vi "Subvi pixel clock.vi"(9 "Line clock":bool) -> (3 "Pixel clock/line clock change":cluster{"Pixel clock":bool, "Line clock":bool})   [LabVIEW 2017]
uses:
  GV N pixel clock per line.vi
  <vilib>/rvi/Memory/Memory_Emulation/nirvimemoryFastEmulation.vi
  <vilib>/rvi/Memory/Memory_Emulation/nirvimemoryEmulation.vi
  <vilib>/rvi/Emulation/niFpgaEmulationIsFPGAContextNoSignature.vi
  <vilib>/rvi/DataTransferAndStorage/Container/Common/niFpgaContainerGetUniqueNameForEmu.vi
  <vilib>/rvi/Emulation/niFpgaProcessEmulError.vi
  <vilib>/rvi/Emulation/niFpgaSctlEmulationGetInTimedLoop.vi
  <vilib>/rvi/errors/nirviReportUnexpectedCaseInternalError (U32).vi
  <vilib>/rvi/DataTransferAndStorage/Container/XNode/niFpgaContainer.xnode
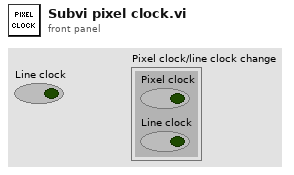
[diagram p1: front panel]
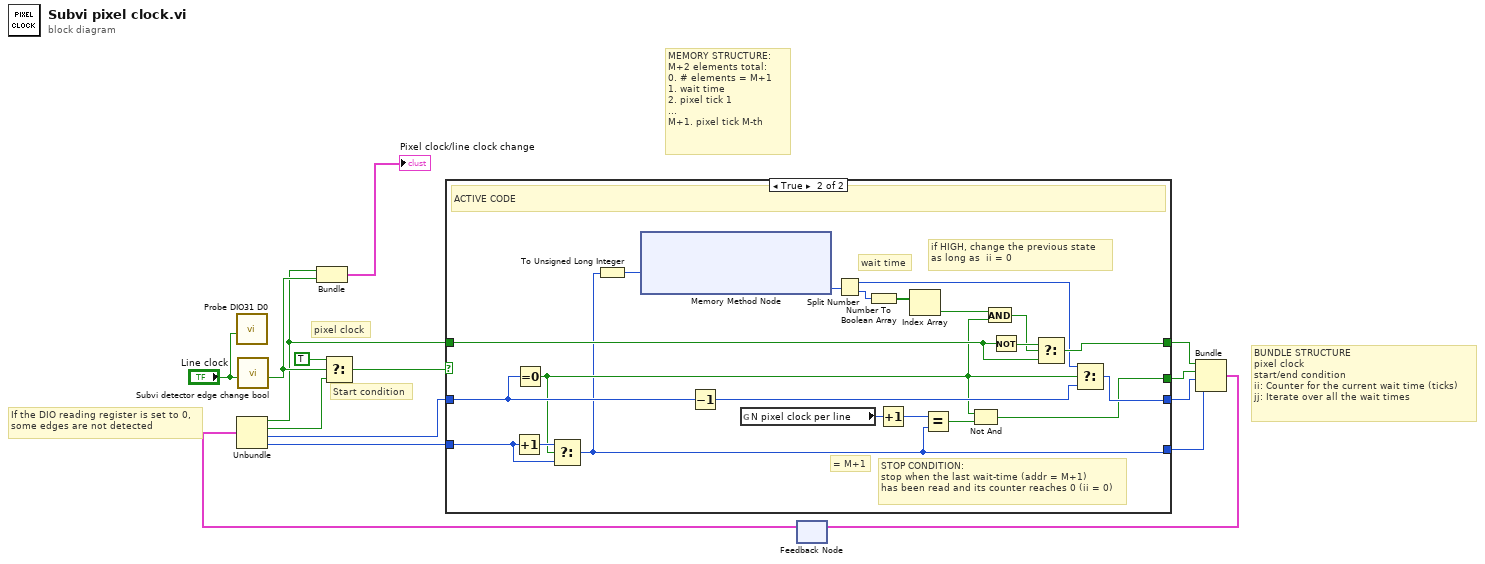
[diagram p0: block diagram]
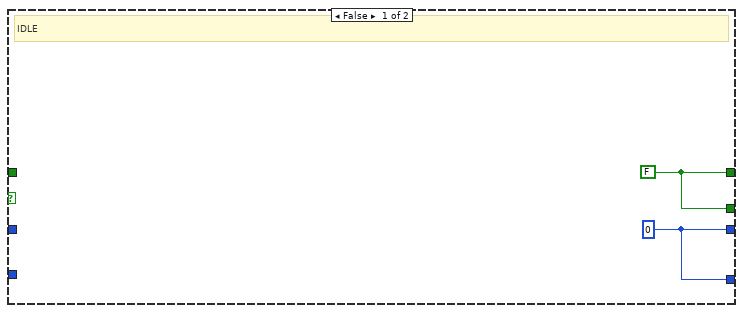
[diagram p2: hidden frame]
diagram:
  # "pixel clock"
  # "If the DIO reading register is set to 0,\nsome edges are not detected"
  # "BUNDLE STRUCTURE\npixel clock\nstart/end condition\nii: Counter for the current wait time (ticks)\njj: Iterate over all the wait times"
  # "MEMORY STRUCTURE:\nM+2 elements total:\n0. # elements = M+1\n1. wait time \n2. pixel tick 1\n...\nM+1. pixel tick M-th"
  # "Start condition"
  n1 = call "Probe DIO31 D0.vi"("D0"="Line clock") -> ()  [unwired: 11 in]
  n2 = call "Subvi detector edge change bool.vi"("Input"="Line clock") -> ("Output"=w3:bool)  [unwired: 8 in]
  n3 = feedback #1() -> (w8:cluster{bool, bool, u16, u16})  [unwired: 1 in]
  n4 = Unbundle(w8) -> (w1:bool, w6:bool, w5:u16, w4:u16)
  n5 = Bundle(w1, "Output"=w3) -> (→"Pixel clock/line clock change":cluster{bool, "Output":bool})  [unwired: 1 in]
  n6 = Select(t=TRUE, s=w3, f=w6) -> (s? t:f=w14:bool)
  n7 = case shown="True" w14 {
    tunnel: [w17 w20] -> w12
    tunnel: w5 -> [_ w30]
    tunnel: [w16 w33] -> w11
    tunnel: [w17 w34] -> w7
    tunnel: w1 -> [_ w31]
    tunnel: w4 -> [_ w29]
    tunnel: [w16 w18] -> w10
    frame False {
      w17 = FALSE
      w16 = u16 0
      # "IDLE"
    }
    frame True {
      # "STOP CONDITION:\nstop when the last wait-time (addr = M+1) \nhas been read and its counter reaches 0 (ii = 0)"
      # "if HIGH, change the previous state\nas long as  ii = 0"
      # "= M+1"
      # "wait time"
      # "ACTIVE CODE"
      n8 = Increment(x=w29) -> (x+1=w38:u16)
      n9 = Equal To 0?(x=w30) -> (x = 0?=w21:bool)
      n10 = Select(t=w38, s=w21, f=w29) -> (s? t:f=w18:u16)
      n11 = To Unsigned Long Integer(number=w18) -> (unsigned 32bit integer=w27:u32)
      n12 = xnode ("Memory Method Node")("Address"=w27) -> ("Data"=w26:u32)  [unwired: 1 in, 1 out]
      n13 = Decrement(x=w30) -> (x-1=w28:u16)
      n14 = global read "GV N pixel clock per line.vi" "N pixel clock per line"() -> (w25:u16)
      n15 = Split Number(x=w26) -> (hi(x)=w32:u16, lo(x)=w36:u16)
      n16 = Number To Boolean Array(number=w36) -> (Boolean array=w37:bool[])
      n17 = Increment(x=w25) -> (x+1=w19:u16)
      n18 = Index Array(array=w37) -> (element=w22:bool)  [unwired: 1 in]
      n19 = Equal?(x=w19, y=w18) -> (x = y?=w24:bool)
      n20 = Not And(1:w24, 2:w21) -> (0:w20:bool)
      n21 = And(x=w22, y=w21) -> (x .and. y?=w23:bool)
      n22 = Not(x=w31) -> (.not. x?=w35:bool)
      n23 = Select(t=w35, s=w23, f=w31) -> (s? t:f=w34:bool)
      n24 = Select(t=w32, s=w21, f=w28) -> (s? t:f=w33:u16)
    }
  }
  n25 = Bundle(w7, w12, w11, w10) -> (w9:cluster{bool, bool, u16, u16})  [unwired: 1 in]
  n26 = feedback-in #1(w9) -> ()
